vi "Grade Individual VI Stats.vi"(8 "Error in":errorcluster caption="Error in (no error)", 9 "Test Config Map":T4 {"Test Config"."Test Ranking" items=["Low", "Normal", "High"]}, 10 "Raw Results":T8[][](array[typedef]), 11 "VI Results":T3) -> (0 "Error out":errorcluster, 3 "Stats by Ranking":T1)   [LabVIEW 2023, in "VIA Results Handling.lvlib"]
doc: "Takes in some parsed VIA Results and transforms them into Stats by Ranking."
uses:
  VIA Results Handling.lvlib
  <vilib>/addons/analyzer/_analyzerctrls.llb/VIAnCtl Results.ctl
  <vilib>/addons/analyzer/_analyzerctrls.llb/VIAnCtl ResultsData (index).ctl
  <vilib>/addons/analyzer/_analyzerctrls.llb/VIAnCtl ResultStatus.ctl
  Test Config Map.ctl
  <vilib>/addons/analyzer/_analyzerctrls.llb/VIAnCtl Test Config Data.ctl
  <vilib>/addons/analyzer/_analyzerctrls.llb/VIAnCtl TestRanking.ctl
  <vilib>/addons/analyzer/_analyzerctrls.llb/VIAnCtl Config Control Value.ctl
  <vilib>/addons/analyzer/_vianresshared.llb/VIAnRes Parsed Results Data (by VI).ctl
  Stats by Ranking.ctl
  Stats Cluster.ctl
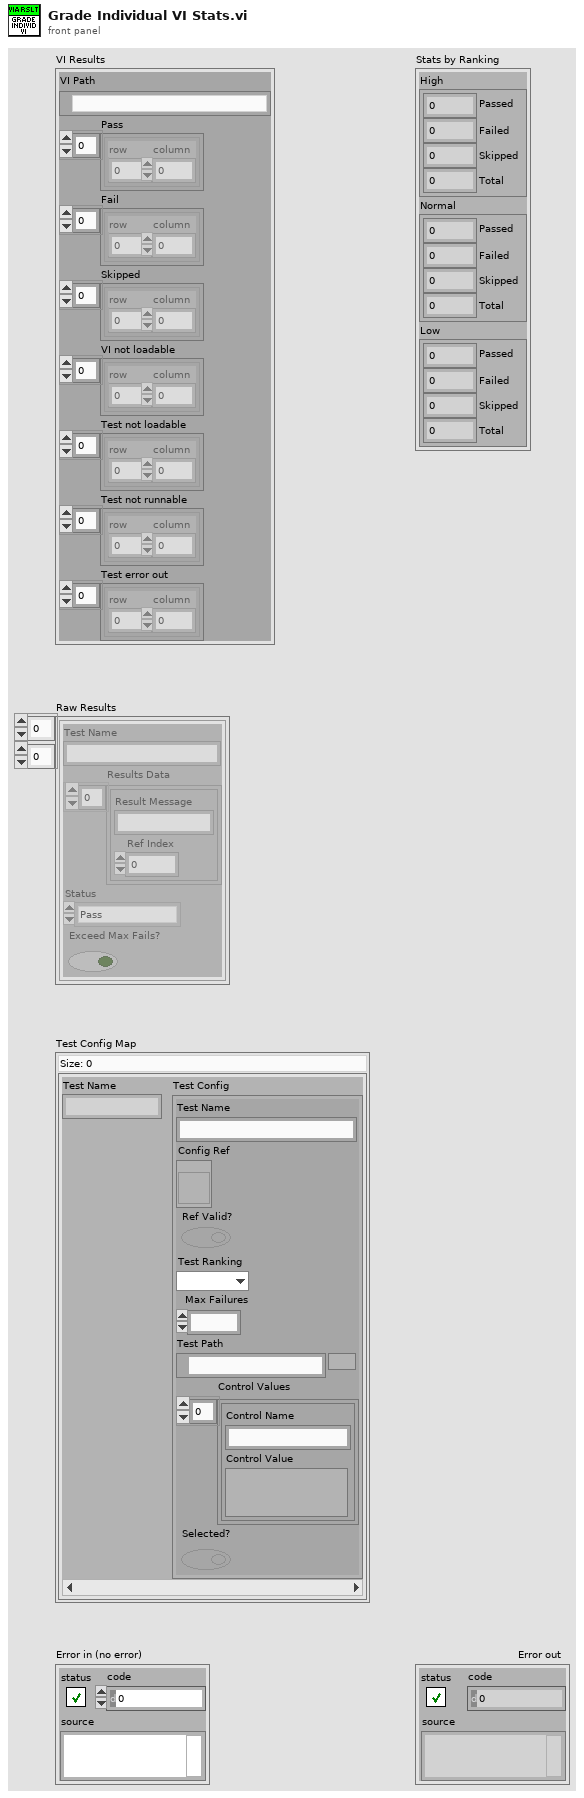
[diagram p1: front panel]
types:
  T1 = typedef "VIA Results Handling.lvlib/Stats by Ranking.ctl" = cluster{"High":T2, "Normal":T2, "Low":T2}
  T2 = typedef "VIA Results Handling.lvlib/Stats Cluster.ctl" = cluster{"Passed":i32, "Failed":i32, "Skipped":i32, "Total":i32}
  T3 = typedef "VIAnRes Parsed Results Data (by VI).ctl" = cluster{"VI Path":path, "Pass":cluster{"row":i32, "column":i32}[], "Fail":cluster{"row":i32, "column":i32}[], "Skipped":cluster{"row":i32, "column":i32}[], "VI not loadable":cluster{"row":i32, "column":i32}[], "Test not loadable":cluster{"row":i32, "column":i32}[], "Test not runnable":cluster{"row":i32, "column":i32}[], "Test error out":cluster{"row":i32, "column":i32}[]}
  T4 = typedef "VIA Results Handling.lvlib/Test Config Map.ctl" = map{string, T5}
  T5 = typedef "VIAnCtl Test Config Data.ctl" = cluster{"Test Name":string, "Config Ref":refnum<vi>, "Ref Valid?":bool, "Test Ranking":T6, "Max Failures":u32, "Test Path":path, "Control Values":T7[], "Selected?":bool}
  T6 = typedef "VIAnCtl TestRanking.ctl" = u16
  T7 = typedef "VIAnCtl Config Control Value.ctl" = cluster{"Control Name":string, "Control Value":variant}
  T8 = typedef "VIAnCtl Results.ctl" = cluster{"Test Name":string, "Results Data":T9[], "Status":T10, "Exceed Max Fails?":bool}
  T9 = typedef "VIAnCtl ResultsData (index).ctl" = cluster{"Result Message":string, "Ref Index":i32}
  T10 = typedef "VIAnCtl ResultStatus.ctl" = enum16{"Pass", "Fail", "Skipped", "VI not loadable", "Test not loadable", "Test not runnable", "Test error out"}
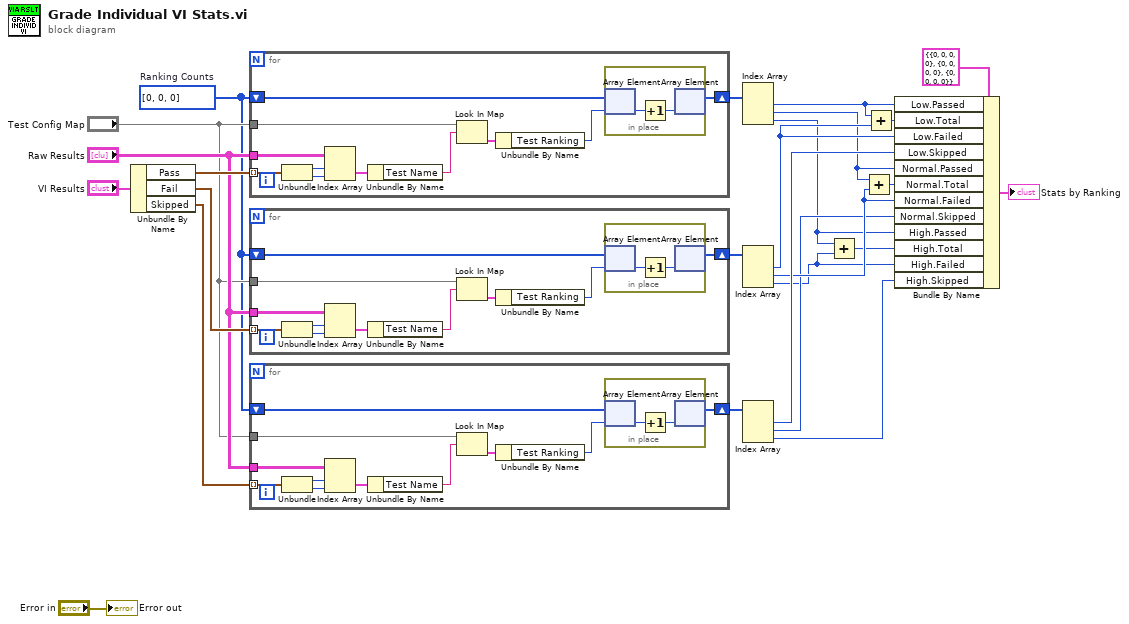
[diagram p0: block diagram]
diagram:
  w19 = i32[] [0, 0, 0]  # Ranking Counts
  n1 = Unbundle By Name("VI Results") -> ("Pass"=w24:cluster{"row":i32, "column":i32}[], "Fail"=w23:cluster{"row":i32, "column":i32}[], "Skipped"=w22:cluster{"row":i32, "column":i32}[])
  n2 = for {
    tunnel: w24 -> [w36] mode=indexing
    tunnel: "Raw Results" -> [w35]
    tunnel: "Test Config Map" -> [w31]
    shift-right: [w26] -> w18
    shift-left: w19 -> [w28]
    n3 = Unbundle(w36) -> ("row"=w34:i32, "column"=w33:i32)
    n4 = Index Array(array=w35, index (row)=w34, index (col)=w33) -> (element=w32:T8)
    n5 = Unbundle By Name(w32) -> ("Test Name"=w30:string)
    n6 = Look In Map(map=w31, key=w30) -> (value=w29:T5)  [unwired: 1 in, 1 out]
    n7 = Unbundle By Name(w29) -> ("Test Ranking"=w27:T6)
    n8 = in-place {
      n9 = in-place-array #1(w28, w27) -> (w38:i32)
      n10 = Increment(x=w38) -> (x+1=w37:i32)
      n11 = in-place-array #1(w37) -> (w26:i32[])  [unwired: 1 out]
    }
  }
  n12 = for {
    tunnel: w23 -> [w49] mode=indexing
    tunnel: "Raw Results" -> [w48]
    tunnel: "Test Config Map" -> [w44]
    shift-right: [w39] -> w17
    shift-left: w19 -> [w41]
    n13 = Unbundle(w49) -> ("row"=w47:i32, "column"=w46:i32)
    n14 = Index Array(array=w48, index (row)=w47, index (col)=w46) -> (element=w45:T8)
    n15 = Unbundle By Name(w45) -> ("Test Name"=w43:string)
    n16 = Look In Map(map=w44, key=w43) -> (value=w42:T5)  [unwired: 1 in, 1 out]
    n17 = Unbundle By Name(w42) -> ("Test Ranking"=w40:T6)
    n18 = in-place {
      n19 = in-place-array #2(w41, w40) -> (w51:i32)
      n20 = Increment(x=w51) -> (x+1=w50:i32)
      n21 = in-place-array #2(w50) -> (w39:i32[])  [unwired: 1 out]
    }
  }
  n22 = for {
    tunnel: w22 -> [w62] mode=indexing
    tunnel: "Raw Results" -> [w61]
    tunnel: "Test Config Map" -> [w57]
    shift-right: [w52] -> w16
    shift-left: w19 -> [w54]
    n23 = Unbundle(w62) -> ("row"=w60:i32, "column"=w59:i32)
    n24 = Index Array(array=w61, index (row)=w60, index (col)=w59) -> (element=w58:T8)
    n25 = Unbundle By Name(w58) -> ("Test Name"=w56:string)
    n26 = Look In Map(map=w57, key=w56) -> (value=w55:T5)  [unwired: 1 in, 1 out]
    n27 = Unbundle By Name(w55) -> ("Test Ranking"=w53:T6)
    n28 = in-place {
      n29 = in-place-array #3(w54, w53) -> (w64:i32)
      n30 = Increment(x=w64) -> (x+1=w63:i32)
      n31 = in-place-array #3(w63) -> (w52:i32[])  [unwired: 1 out]
    }
  }
  n32 = Index Array(array=w18) -> (element #1=w14:i32, element #2=w9:i32, element #3=w5:i32)  [unwired: 3 in]
  n33 = Index Array(array=w17) -> (element #1=w13:i32, element #2=w8:i32, element #3=w4:i32)  [unwired: 3 in]
  n34 = Index Array(array=w16) -> (element #1=w15:i32, element #2=w6:i32, element #3=w2:i32)  [unwired: 3 in]
  n35 = Add(x=w5, y=w4) -> (x+y=w3:i32)
  n36 = Add(x=w9, y=w8) -> (x+y=w7:i32)
  n37 = Add(x=w14, y=w13) -> (x+y=w12:i32)
  n38 = Bundle By Name(cluster=T1 {"High"={"Passed"=0, "Failed"=0, "Skipped"=0, "Total"=0}, "Normal"={"Passed"=0, "Failed"=0, "Skipped"=0, "Total"=0}, "Low"={"Passed"=0, "Failed"=0, "Skipped"=0, "Total"=0}} ("Stats by Ranking"), "Low.Passed"=w14, "Low.Total"=w12, "Low.Failed"=w13, "Low.Skipped"=w15, "Normal.Passed"=w9, "Normal.Total"=w7, "Normal.Failed"=w8, "Normal.Skipped"=w6, "High.Passed"=w5, "High.Total"=w3, "High.Failed"=w4, "High.Skipped"=w2) -> (→"Stats by Ranking":T1)
  "Error out" <- "Error in"
